vi "CorrectResponse.vi"(8 "error in (no error)":errorcluster, 11 "TrialBasedExperiment in":refnum<class "WhiteNoiseOrientationDetection.lvclass">) -> (0 "error out":errorcluster, 3 "TrialBasedExperiment out":refnum<class "WhiteNoiseOrientationDetection.lvclass">)   [LabVIEW 2014, in "WhiteNoiseOrientationDetection.lvclass"]
uses:
  WhiteNoiseOrientationDetection.lvclass
  WhiteNoiseOrientationDetection.lvclass/WhiteNoiseOrientationDetection.ctl
  Trial Based Experiment Statechart/MatlabExperiment/MatlabExperiment.lvclass
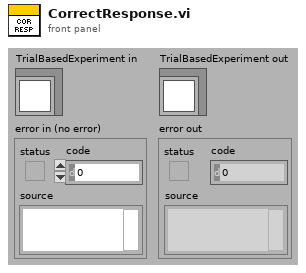
[diagram p1: front panel]
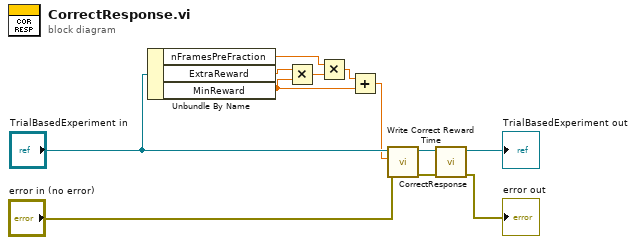
[diagram p0: block diagram]
diagram:
  n1 = Unbundle By Name("TrialBasedExperiment in") -> ("nFramesPreFraction"=w1:dbl, "ExtraReward"=w2:dbl, "MinReward"=w5:dbl)
  n2 = Multiply(x=w2, y=w5) -> (x*y=w4:dbl)
  n3 = Multiply(x=w1, y=w4) -> (x*y=w11:dbl)
  n4 = Add(x=w11, y=w5) -> (x+y=w3:dbl)
  n5 = call-dynamic "Write Correct Reward Time.vi"("error in (no error)"="error in (no error)", "Correct Reward Time"=w3, "MatlabExperiment in"="TrialBasedExperiment in") -> ("error out"=w7:errorcluster, "MatlabExperiment out"=w10:refnum<class "WhiteNoiseOrientationDetection.lvclass">)  [unwired: 7 in]
  n6 = call-parent "CorrectResponse.vi"("error in (no error)"=w7, "TrialBasedExperiment in"=w10) -> ("error out"=→"error out":errorcluster, "TrialBasedExperiment out"=→"TrialBasedExperiment out":refnum<class "WhiteNoiseOrientationDetection.lvclass">)  [unwired: 8 in]
